vi "Get Plugin Node.vi"(8 "error in (no error)":errorcluster, 11 "Item Ref in":T1 format="%.0x") -> (0 "error out":errorcluster, 1 "found?":bool, 2 "Plugin Ref":T1 format="%.0x", 3 "Item Ref out":T1 format="%.0x")   [LabVIEW 2020, in "DSF System Explorer.lvlib"]
uses:
  DSF System Explorer.lvlib
  <vilib>/NI VeriStand/Custom Device API/Custom Device Item Ref.ctl
  Shared/Plugin Page GUID.vi
  <vilib>/NI VeriStand/Custom Device API/Custom Device API.lvlib
  Shared/DSF Shared.lvlib
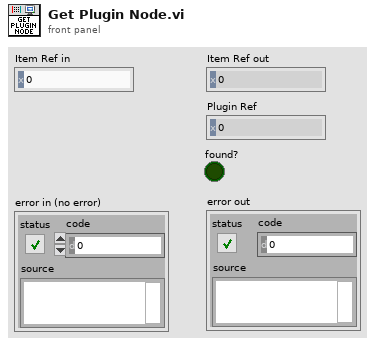
[diagram p1: front panel]
types:
  T1 = typedef "Custom Device API.lvlib/Custom Device Item Ref.ctl" = u64
  T2 = typedef "Custom Device API.lvlib/Custom Device Item Info.ctl" = cluster{"Name":string, "Is Channel":bool, "GUID":string, "Is Waveform":bool}
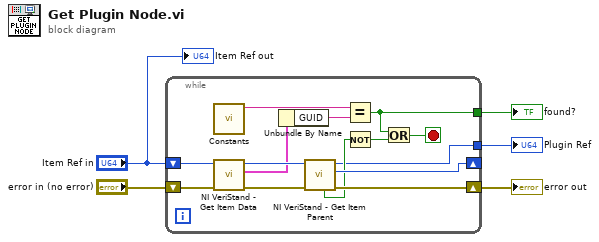
[diagram p0: block diagram]
diagram:
  n1 = while {
    shift-right: [w13] -> w3
    shift-left: "error in (no error)" -> [w16]
    shift-right: [w12] -> _
    shift-left: "Item Ref in" -> [w17]
    tunnel: [w9] -> w2
    tunnel: [w6] -> w1
    stop <- w7 stop-if-true
    n2 = call-poly "Constants.vi"() -> ("Plugin GUID"=w19:string)  [unwired: 11 in]
    n3 = call <vilib>:"NI VeriStand - Get Item Data.vi"("error in (no error)"=w16, "Item Ref in"=w17) -> ("error out"=w11:errorcluster, "Item Info"=w14:T2, "Item Ref out"=w15:T1)  [unwired: 6 in, 1 out]
    n4 = Unbundle By Name(w14) -> ("GUID"=w18:string)
    n5 = call <vilib>:"NI VeriStand - Get Item Parent.vi"("error in (no error)"=w11, "Item Ref in"=w15) -> ("error out"=w13:errorcluster, "Parent Ref"=w12:T1, "Item Ref out"=w9:T1, "Found"=w10:bool)  [unwired: 6 in]
    n6 = Equal?(x=w19, y=w18) -> (x = y?=w6:bool)
    n7 = Not(x=w10) -> (.not. x?=w8:bool)
    n8 = Or(x=w6, y=w8) -> (x .or. y?=w7:bool)
  }
  "error out" <- w3
  "Plugin Ref" <- w2
  "found?" <- w1
  "Item Ref out" <- "Item Ref in"
